vi "CreatNouvChampHeader.vi"(9 "CommentairChamp":string, 10 "ValChamp":string, 11 "NomChamp":string="toto") -> (3 "ChampHeader":string)   [LabVIEW 2020]
panel:
  out "substring":string
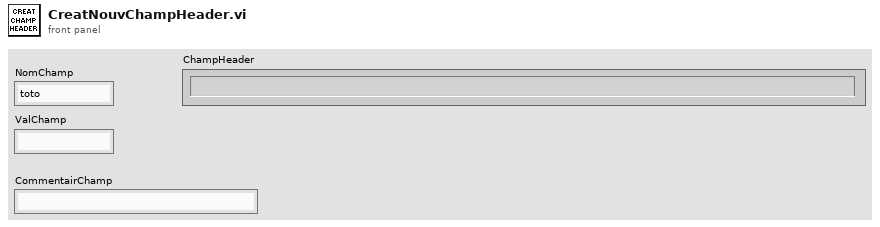
[diagram p1: front panel]
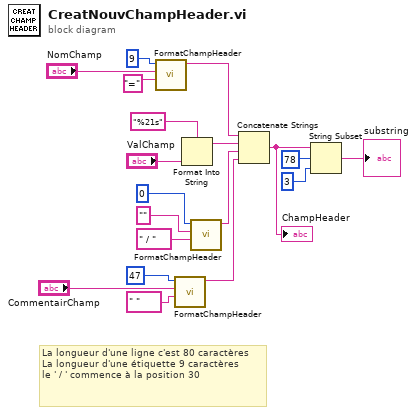
[diagram p0: block diagram]
diagram:
  # "La longueur d'une ligne c'est 80 caractères\nLa longueur d'une étiquette 9 caractères\nle ' / ' commence à la position 30"
  n1 = call "FormatChampHeader.vi"("Caractère"="=", "NomChamp"="NomChamp", "Longueur"=9) -> ("String"=w4:string)  [unwired: 8 in]
  n2 = call "FormatChampHeader.vi"("Caractère"=" ", "NomChamp"="CommentairChamp", "Longueur"=47 ("Longueur 3")) -> ("String"=w8:string)  [unwired: 8 in]
  n3 = Format Into String(format string="%21s", "ValChamp") -> (resulting string=w3:string)  [unwired: 2 in, 1 out]
  n4 = call "FormatChampHeader.vi"("Caractère"=" / ", "NomChamp"="", "Longueur"=0 ("Longueur 2")) -> ("String"=w14:string)  [unwired: 8 in]
  n5 = Concatenate Strings(w4, w3, w14, w8) -> (w6:string)
  "ChampHeader" <- w6
  n6 = String Subset(string=w6, offset (0)=78, length (rest)=3 ("length (rest)")) -> (substring=→"substring":string)
